vi "Script to Graph.vi"(0 "Script":T1, 5 "tr":dbl=1.0) -> (4 "XY Data":cluster{"X":dbl[], "Y":dbl[]}[](array[cluster]))   [LabVIEW 2019]
uses:
  TypeDef/Script.ctl
  TypeDef/Step.ctl
  TypeDef/Direction.ctl
panel:
  out "XY Graph":cluster{dbl[], dbl[]}[](graph)
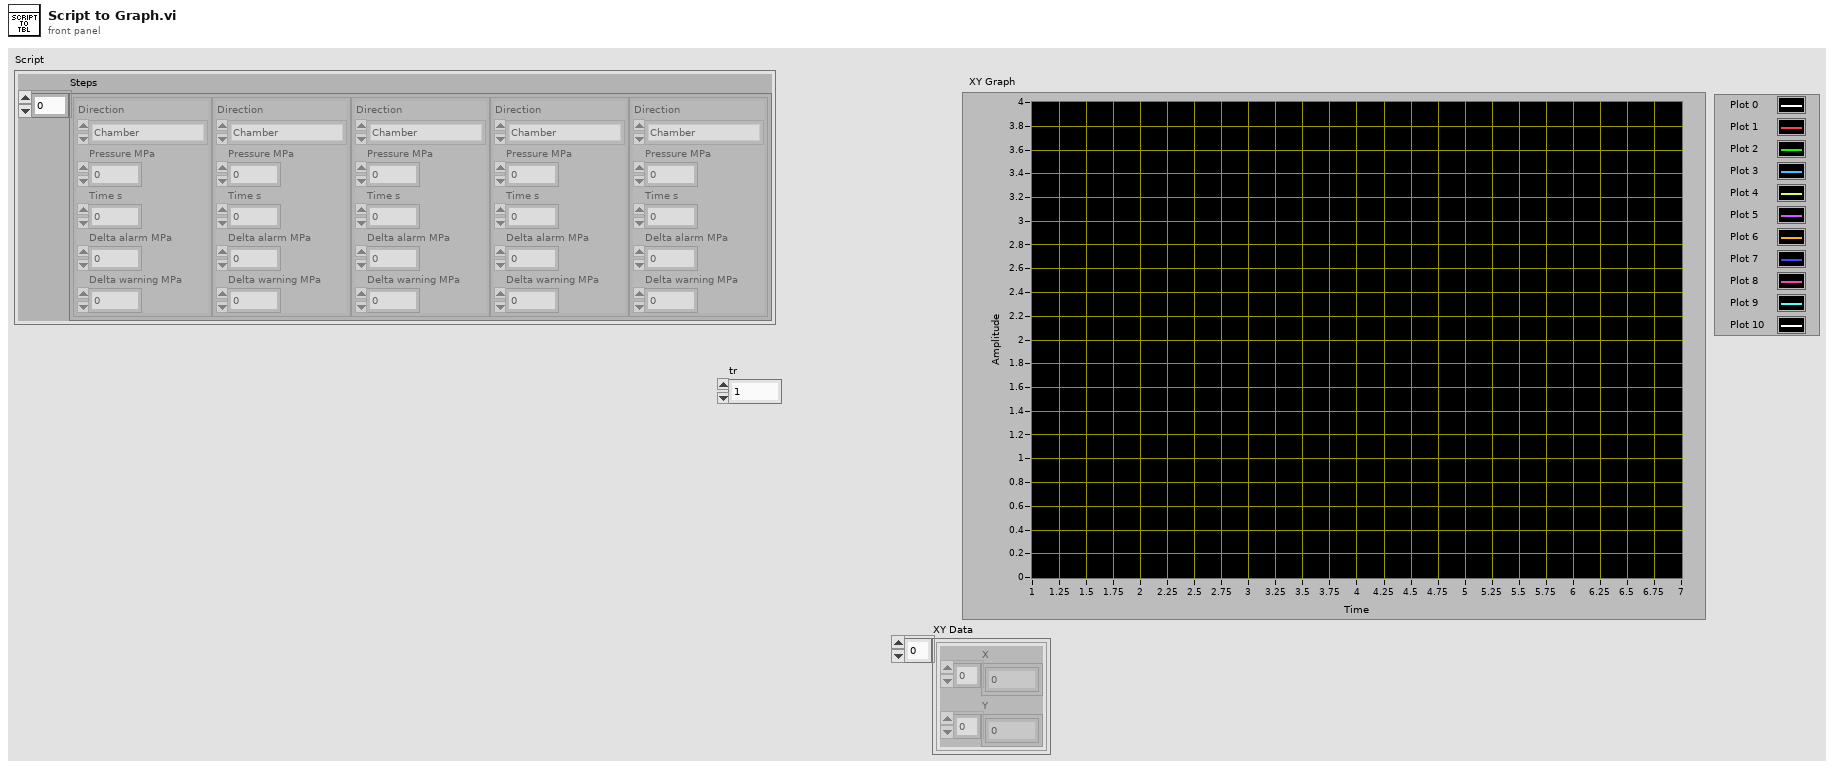
[diagram p1: front panel]
types:
  T1 = typedef "Script.ctl" = cluster{"Steps":T2[]}
  T2 = typedef "Step.ctl" = cluster{"Direction":T3, "Pressure MPa":dbl, "Time s":dbl, "Delta alarm MPa":dbl, "Delta warning MPa":dbl}
  T3 = typedef "Direction.ctl" = enum16{"DUT", "Chamber"}
  T4 = cluster{"P Chamber":dbl, "P Chamber A":dbl, "P Chamber W":dbl, "P DUT":dbl, "P DUT A":dbl, "P DUT W":dbl, "TIME":dbl}
  T5 = cluster{"P Chamber":dbl, "P Chamber A":dbl, "P Chamber W":dbl, "P DUT":dbl, "P DUT A":dbl, "P DUT W":dbl, "TIME":dbl}[]
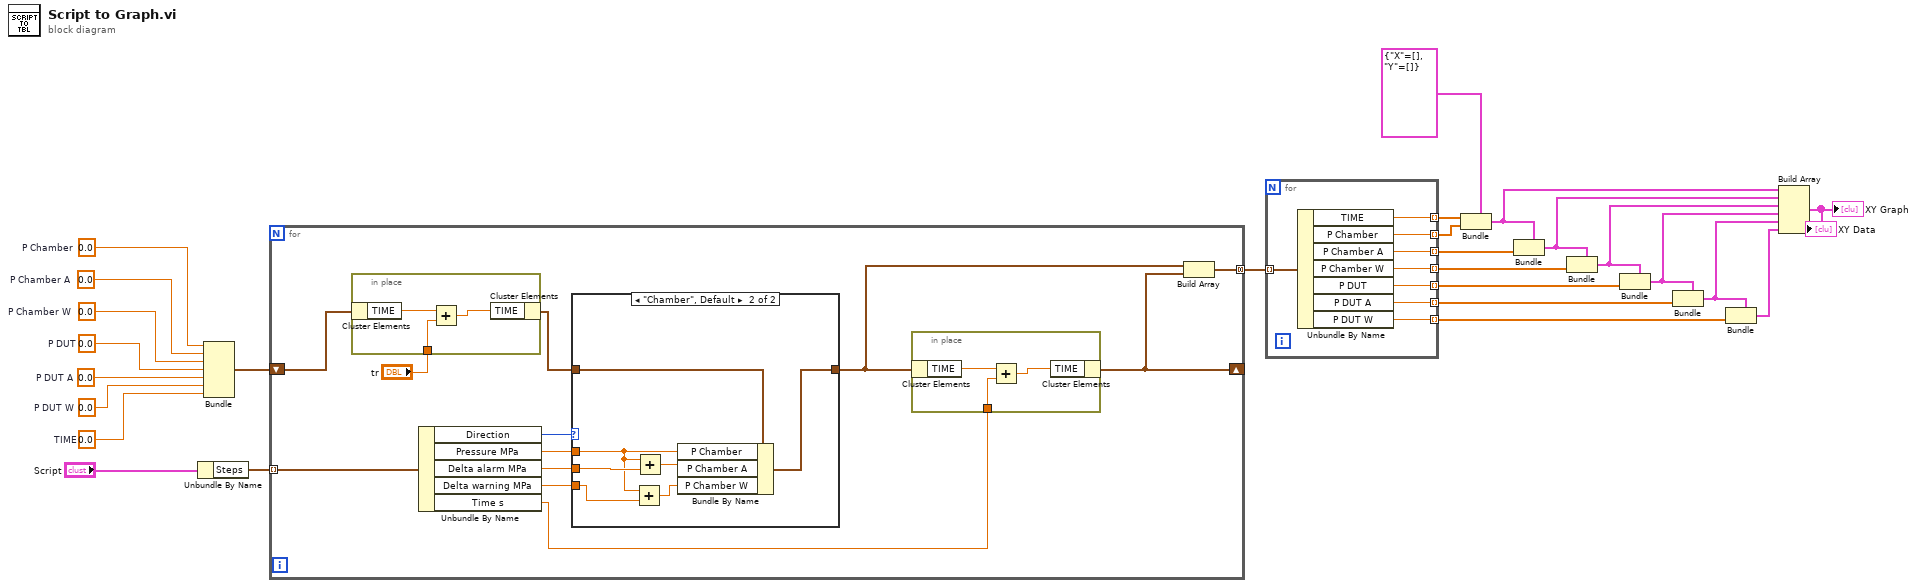
[diagram p0: block diagram]
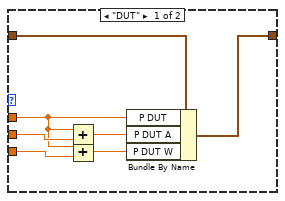
[diagram p2: hidden frame]
diagram:
  w17 = 0.0  # TIME
  w19 = 0.0  # P DUT W
  w22 = 0.0  # P Chamber W
  w20 = 0.0  # P DUT A
  w23 = 0.0  # P Chamber A
  w21 = 0.0  # P DUT
  w24 = 0.0  # P Chamber
  n1 = Unbundle By Name("Script") -> ("Steps"=w25:T2[])
  n2 = Bundle("P Chamber"=w24, "P Chamber A"=w23, "P Chamber W"=w22, "P DUT"=w21, "P DUT A"=w20, "P DUT W"=w19, "TIME"=w17) -> (w18:T4)  [unwired: 1 in]
  n3 = for {
    tunnel: w25 -> [w38] mode=indexing
    shift-right: [w31] -> _
    shift-left: w18 -> [w29]
    tunnel: [w33] -> w16 mode=concatenating
    n4 = in-place {
      in-place-border: "tr" -> [w39]
      n5 = in-place-cluster #1(w29) -> ("TIME"=w41:dbl)
      n6 = Add(x=w41, y=w39) -> (x+y=w40:dbl)
      n7 = in-place-cluster #1("TIME"=w40) -> (w28:T4)
    }
    n8 = Unbundle By Name(w38) -> ("Direction"=w37:T3, "Pressure MPa"=w36:dbl, "Delta alarm MPa"=w35:dbl, "Delta warning MPa"=w34:dbl, "Time s"=w30:dbl)
    n9 = case shown="\"Chamber\", Default" w37 {
      tunnel: w28 -> [w51 w58]
      tunnel: w36 -> [w47 w53]
      tunnel: w35 -> [w49 w57]
      tunnel: w34 -> [w48 w54]
      tunnel: [w50 w56] -> w32
      frame "DUT" {
        n10 = Add(x=w47, y=w49) -> (x+y=w46:dbl)
        n11 = Add(x=w47, y=w48) -> (x+y=w45:dbl)
        n12 = Bundle By Name(cluster=w51, "P DUT"=w47, "P DUT A"=w46, "P DUT W"=w45) -> (w50:T4)
      }
      frame "Chamber", Default {
        n13 = Add(x=w53, y=w54) -> (x+y=w52:dbl)
        n14 = Add(x=w53, y=w57) -> (x+y=w55:dbl)
        n15 = Bundle By Name(cluster=w58, "P Chamber"=w53, "P Chamber A"=w55, "P Chamber W"=w52) -> (w56:T4)
      }
    }
    n16 = in-place {
      in-place-border: w30 -> [w42]
      n17 = in-place-cluster #2(w32) -> ("TIME"=w44:dbl)
      n18 = Add(x=w44, y=w42) -> (x+y=w43:dbl)
      n19 = in-place-cluster #2("TIME"=w43) -> (w31:T4)
    }
    n20 = Build Array(w32, w31) -> (w33:T5)
  }
  n21 = for {
    tunnel: w16 -> [w66] mode=indexing
    tunnel: [w65] -> w15 mode=indexing
    tunnel: [w64] -> w14 mode=indexing
    tunnel: [w63] -> w13 mode=indexing
    tunnel: [w62] -> w12 mode=indexing
    tunnel: [w61] -> w11 mode=indexing
    tunnel: [w60] -> w10 mode=indexing
    tunnel: [w59] -> w9 mode=indexing
    n22 = Unbundle By Name(w66) -> ("TIME"=w65:dbl, "P Chamber"=w64:dbl, "P Chamber A"=w63:dbl, "P Chamber W"=w62:dbl, "P DUT"=w61:dbl, "P DUT A"=w60:dbl, "P DUT W"=w59:dbl)
  }
  n23 = Bundle(cluster=cluster{"X":dbl[], "Y":dbl[]} {"X"=[], "Y"=[]}, "X"=w15, "Y"=w14) -> (w8:cluster{"X":dbl[], "Y":dbl[]})
  n24 = Bundle(cluster=w8, "Y"=w13) -> (w7:cluster{"X":dbl[], "Y":dbl[]})  [unwired: 1 in]
  n25 = Bundle(cluster=w7, "Y"=w12) -> (w6:cluster{"X":dbl[], "Y":dbl[]})  [unwired: 1 in]
  n26 = Bundle(cluster=w6, "Y"=w11) -> (w5:cluster{"X":dbl[], "Y":dbl[]})  [unwired: 1 in]
  n27 = Bundle(cluster=w5, "Y"=w10) -> (w4:cluster{"X":dbl[], "Y":dbl[]})  [unwired: 1 in]
  n28 = Bundle(cluster=w4, "Y"=w9) -> (w3:cluster{"X":dbl[], "Y":dbl[]})  [unwired: 1 in]
  n29 = Build Array(w8, w7, w6, w5, w4, w3) -> (→"XY Graph" →"XY Data":cluster{"X":dbl[], "Y":dbl[]}[])
